vi "Math.Calculate, Vrms to Vp and Vpp.vi"(3 "Vrms":dbl) -> (0 "Vpeak":dbl, 1 "Vpp":dbl)   [LabVIEW 2024, in "EQMF.lvlib" / "Math Utils.lvlib"]
uses:
  Math Utils.lvlib
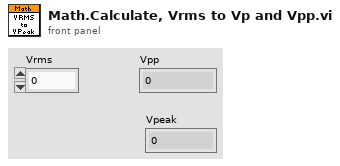
[diagram p1: front panel]
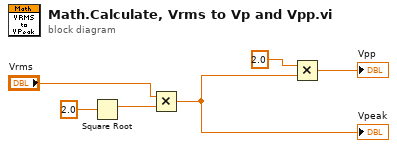
[diagram p0: block diagram]
diagram:
  n1 = Square Root(x=2.0) -> (sqrt(x)=w5:dbl)
  n2 = Multiply(x="Vrms", y=w5) -> (x*y=w2:dbl)
  "Vpeak" <- w2
  n3 = Multiply(x=2.0, y=w2) -> (x*y=→"Vpp":dbl)
